vi "Dashboard Main.vi"() -> ()   [LabVIEW 2023]
uses:
  52f2dcef-b32f-41dc-9262-467f65fbdc6c.vi
  <vilib>/Rock Robotics/Network Tables/NT Write String Array.vi
  <vilib>/Rock Robotics/WPI/Dashboard/WPI_DashboardLogging Global.vi
  <vilib>/Rock Robotics/Network Tables/NT Write Boolean.vi
panel:
  in  "Camera Settings Right":T1={"Frame Rate"=30, "Compression"=30, "Size"=1, "DB Camera Config"=FALSE} {"Frame Rate" scale=1.0..30.0; "Compression" scale=100.0..-1.0; "Size" items=["640x480", "320x240", "160x120"]}
  in  "Camera Name Right":string(combo)="No Camera Selection"
  out "NT Connection":bool
  in  "Camera Settings":T1={"Frame Rate"=30, "Compression"=30, "Size"=1, "DB Camera Config"=FALSE} {"Frame Rate" scale=1.0..30.0; "Compression" scale=100.0..-1.0; "Size" items=["640x480", "320x240", "160x120"]}
  in  "Camera Name":string(combo)="No Camera Selection"
  in  "TCP":refnum<k5>
  in  "Rec Mode":enum32{"Stop", "Record", "Playback"}(radio)
  out "Robot IP":string
  out "Image Message":string="Timeout in Camera Communications"
  in  "Dashboard Tab":T2(tab)
  in  "Auto Type":string
  out "Match Safe?":bool
  out "Cascade Level":string
  in  "Auto Delay?":bool
  in  "Delay Time (s)":dbl
  out "E.E. Setpoint":dbl
  in  "Aquitaine File":string
  in  "Climb Arm Reset":bool
  out "Intake Setpoint":dbl
  in  "Auto Calibrate":bool=TRUE
  in  "Robot Selector":u16(ring) items=["2468 Competition", "2468 Practice"]
  in  "Manual Paths":string[](array[string])
  in  "Max Rotation":dbl=400.0
  in  "Max Translation":dbl=19.0
  in  "Deadband":dbl=0.05
  in  "Auto Selector":T3(ring)
  out "IMU":dbl(knob) scale=-180.0..180.0
  in  "Select Auto":string(combo)="Select Autonomous ..."
  out "Mode":T4(ring)=enum."Auto Disabled"
  out "Camera Perf":cluster{"Bandwidth (Mbps)":dbl, "FPS":dbl}
  out "Cascade Sensor":dbl
  out "Camera Perf 2":string
  out "Auto Picture":picture
  out "Cascade State":string
  out "Has Coral?":string
  out "Algae State":string
  out "Climb State":string
  in  "Amp Scale":dbl=0.97
  out "Shooter Hood":dbl
  out "Distance from Speaker":dbl
  out "Trap Auto Align":bool
  out "Camera Image Right":T5(plugin-control)
  out "Speaker Auto Align":bool
  out "Field Centric":bool
  out "Camera Image":T5(plugin-control)
  out "Current Shot":T6(ring)
  out "In Range?":bool
  out "Tree":string(tree)
  # "HW"
  # "HW"
  # "IMU"
  # "SWERVE"
  # "AUTONOMOUS"
  # "CONFIGS"
  # "FEEDBACK"
  # "INTAKE VIEW"
  # "SHOOTER VIEW"
  # "FIELD CENTRIC"
  # "SPEAKER AA"
  # "TRAP AA"
  # "CAN ERROR"
  # "SENSOR FAULT"
  # "GATE DRIVER"
  # "No POWER"
  # "FuLL FORWARD"
  # "FuLL REVERSE"
  # "BRUSHED BRAKE"
  # "BRUSHED COAST"
  # "BRUSHLESS BRAKE"
  # "BRUSHLESS COAST"
  # "RECOVERY MODE/OFF"
  # "https://cdn8.bigcommerce.com/s-t3eo8vwp22/product_images/uploaded_images/fault-no-12v.gif"
  # "PIGEON 2"
  # "DAMAGED HARDWARE"
  # "BOOTLOADER"
  # "CAN FAULT"
  # "ROBOT DISABLED"
  # "ROBOT ENABLED"
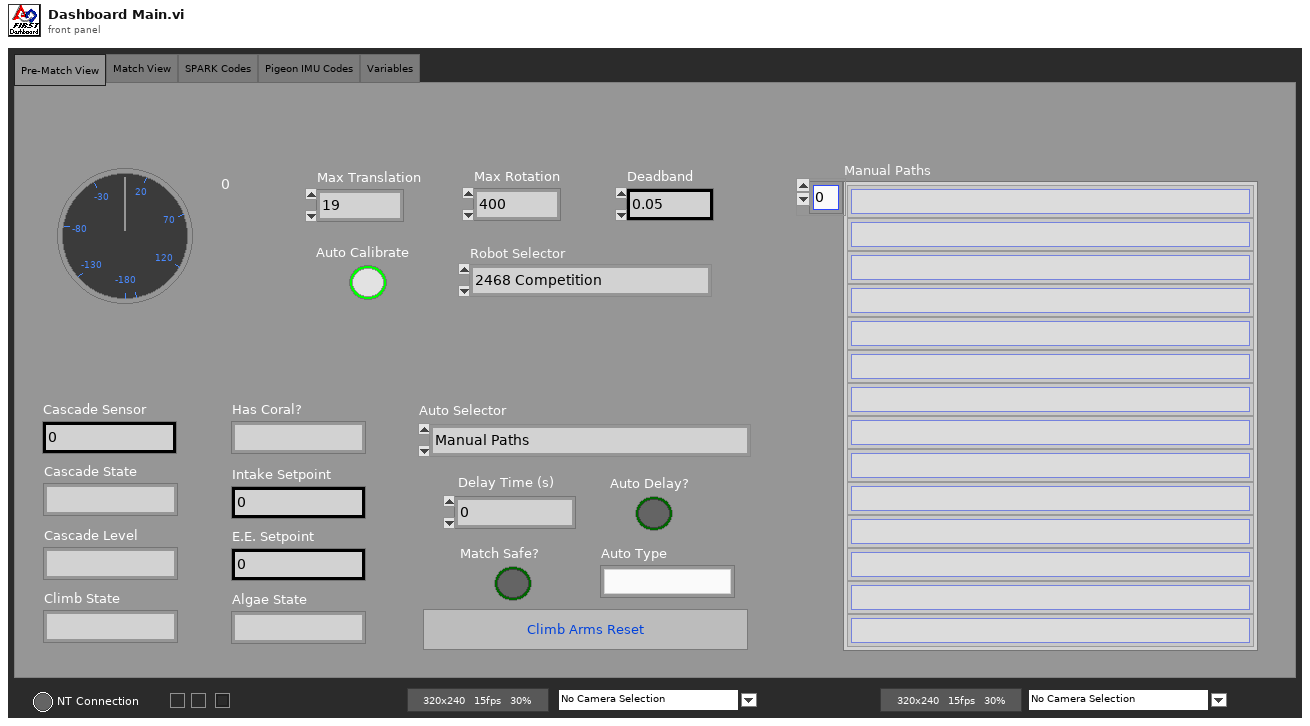
[diagram p1: front panel]
types:
  T1 = cluster{"Frame Rate":i32, "Compression":i32, "Size":u16, "DB Camera Config":bool}
  T2 = enum32{"Pre-Match View", "Match View", "SPARK Codes", "Pigeon IMU Codes", "Variables"}
  T3 = enum16{"Manual Paths", "Reef Align Auto", "1 High Coral Left Side", "1 High Coral Center (SAFE)"}
  T4 = enum8{"Tele-Op Disabled", "Tele-Op Enabled", "Auto Disabled", "Auto Enabled", "Test Disabled", "Test Enabled", "Disconnected", "No Code", "E-Stop"}
  T5 = typedef "IMAQ Image.ctl" = refnum<image>
  T6 = enum32{"Soft Lob", "Amp", "Subwoofer", "Long Lob", "Idle", "Zero", "Trap", "Interpolation"}
  T7 = cluster{"Save Path":path, "Interval (s)":dbl, "Keep":i32}
  T8 = typedef "Image Type" = u32
  T9 = enum32{"Pre-Match View", "Match View", "SparkMax Codes", "Pigeon IMU Codes", "Variables"}
  T10 = cluster{"IDs":cluster{"RPC field ID":u16, "Unique ID":u16}, "String":string}
  T11 = cluster{"Dashboard Tab":refnum<vi>, "Rec Mode":refnum<vi>, "Tree":refnum<vi>, "Camera Perf 2":refnum<vi>, "Camera Settings":refnum<vi>, "Camera Name":refnum<vi>, "Camera Image":refnum<vi>}
  T12 = cluster{"Global Rectangle":i32[], "Contours":cluster{"Contour Type":u32, "ROI Type":u32, "Points":i32[]}[]}
  T13 = cluster{"Camera Name Right":string, string, "Saved DB Images Info":cluster{"Save Path":path, "Interval (s)":dbl, "Keep":i32}}
  T14 = cluster{"Camera Name":string, string, "Saved DB Images Info":cluster{"Save Path":path, "Interval (s)":dbl, "Keep":i32}}
  T15 = cluster{"Error Strings":string, "Disable Counts":cluster{u16, u16}, "Rail Faults":cluster{u16, u16, u16}, "Robot IP":string, "DB Mode":u8, "Event Info":cluster{"Name":string, "Type":u8, "Number":u16, "Replay":u8}}
  T16 = cluster{"Storage":cluster{"Disk Free":u64, "RAM Block":u32, "RAM free":u32}, "CPU Utilization":cluster{"CPU % ISR":sgl, "CPU % Time Crit":sgl, "CPU % Timed Str":sgl, "CPU % High":sgl, "CPU % Above":sgl, "CPU % Normal":sgl, "CPU % Low":sgl}, "CAN":cluster{"% Bus Utilization":sgl, "Bus Off Cnt":u32, "TX_FIFO Full Cnt":u32, "Receive Error Cnt":u8, "Transmit Error Cnt":u8}, "HID":cluster{"HID Outputs":u32, "Rumble Low":u16, "Rumble High":u16}[]}
  T17 = cluster{"Status bits":cluster{"Test Mode":bool, "Autonomous":bool, "Enabled":bool, "Code Start":bool, "Brownout":bool, "Reserved 2":bool, "Reserved 3":bool, "E-Stop":bool}, "Code Trace":cluster{"Disabled":bool, "TeleOp":bool, "Auto":bool, "Test":bool}, "Controller Type":enum16{"unknown", "cRIO", "roboRio"}, "Code?":enum16{"unknown", "noCode", "code"}, "Battery V":dbl}
  T18 = cluster{"Control Bits":cluster{"TestMode":bool, "Autonomous":bool, "Enabled":bool, "FMS Present":bool, bool, bool, bool, "E-Stop":bool}, "Team Station ":u8, "Countdown":sgl, "Joystick Values":cluster{"Axes":dbl[], "Buttons":bool[], "POVs":i16[]}[]}
  T19 = typedef "imagedata.ctl" = cluster{"image type":i32, "image depth":i32, "image":u8[], "mask":u8[], "colors":u32[], "Rectangle":cluster{"left":i16, "top":i16, "right":i16, "bottom":i16}}
  T20 = cluster{"Operation":enum16{"Update", "Clear"}, "Color Box":u32}[]
  T21 = cluster{"Image Size":bool, "Image Type":bool, "Pixel Value":bool, "ROI Information":bool, "Zoom Factor":bool}
  T22 = cluster{"Shift":bool, "Ctrl":bool, "Alt":bool, "Cmd":bool, "Opt":bool}
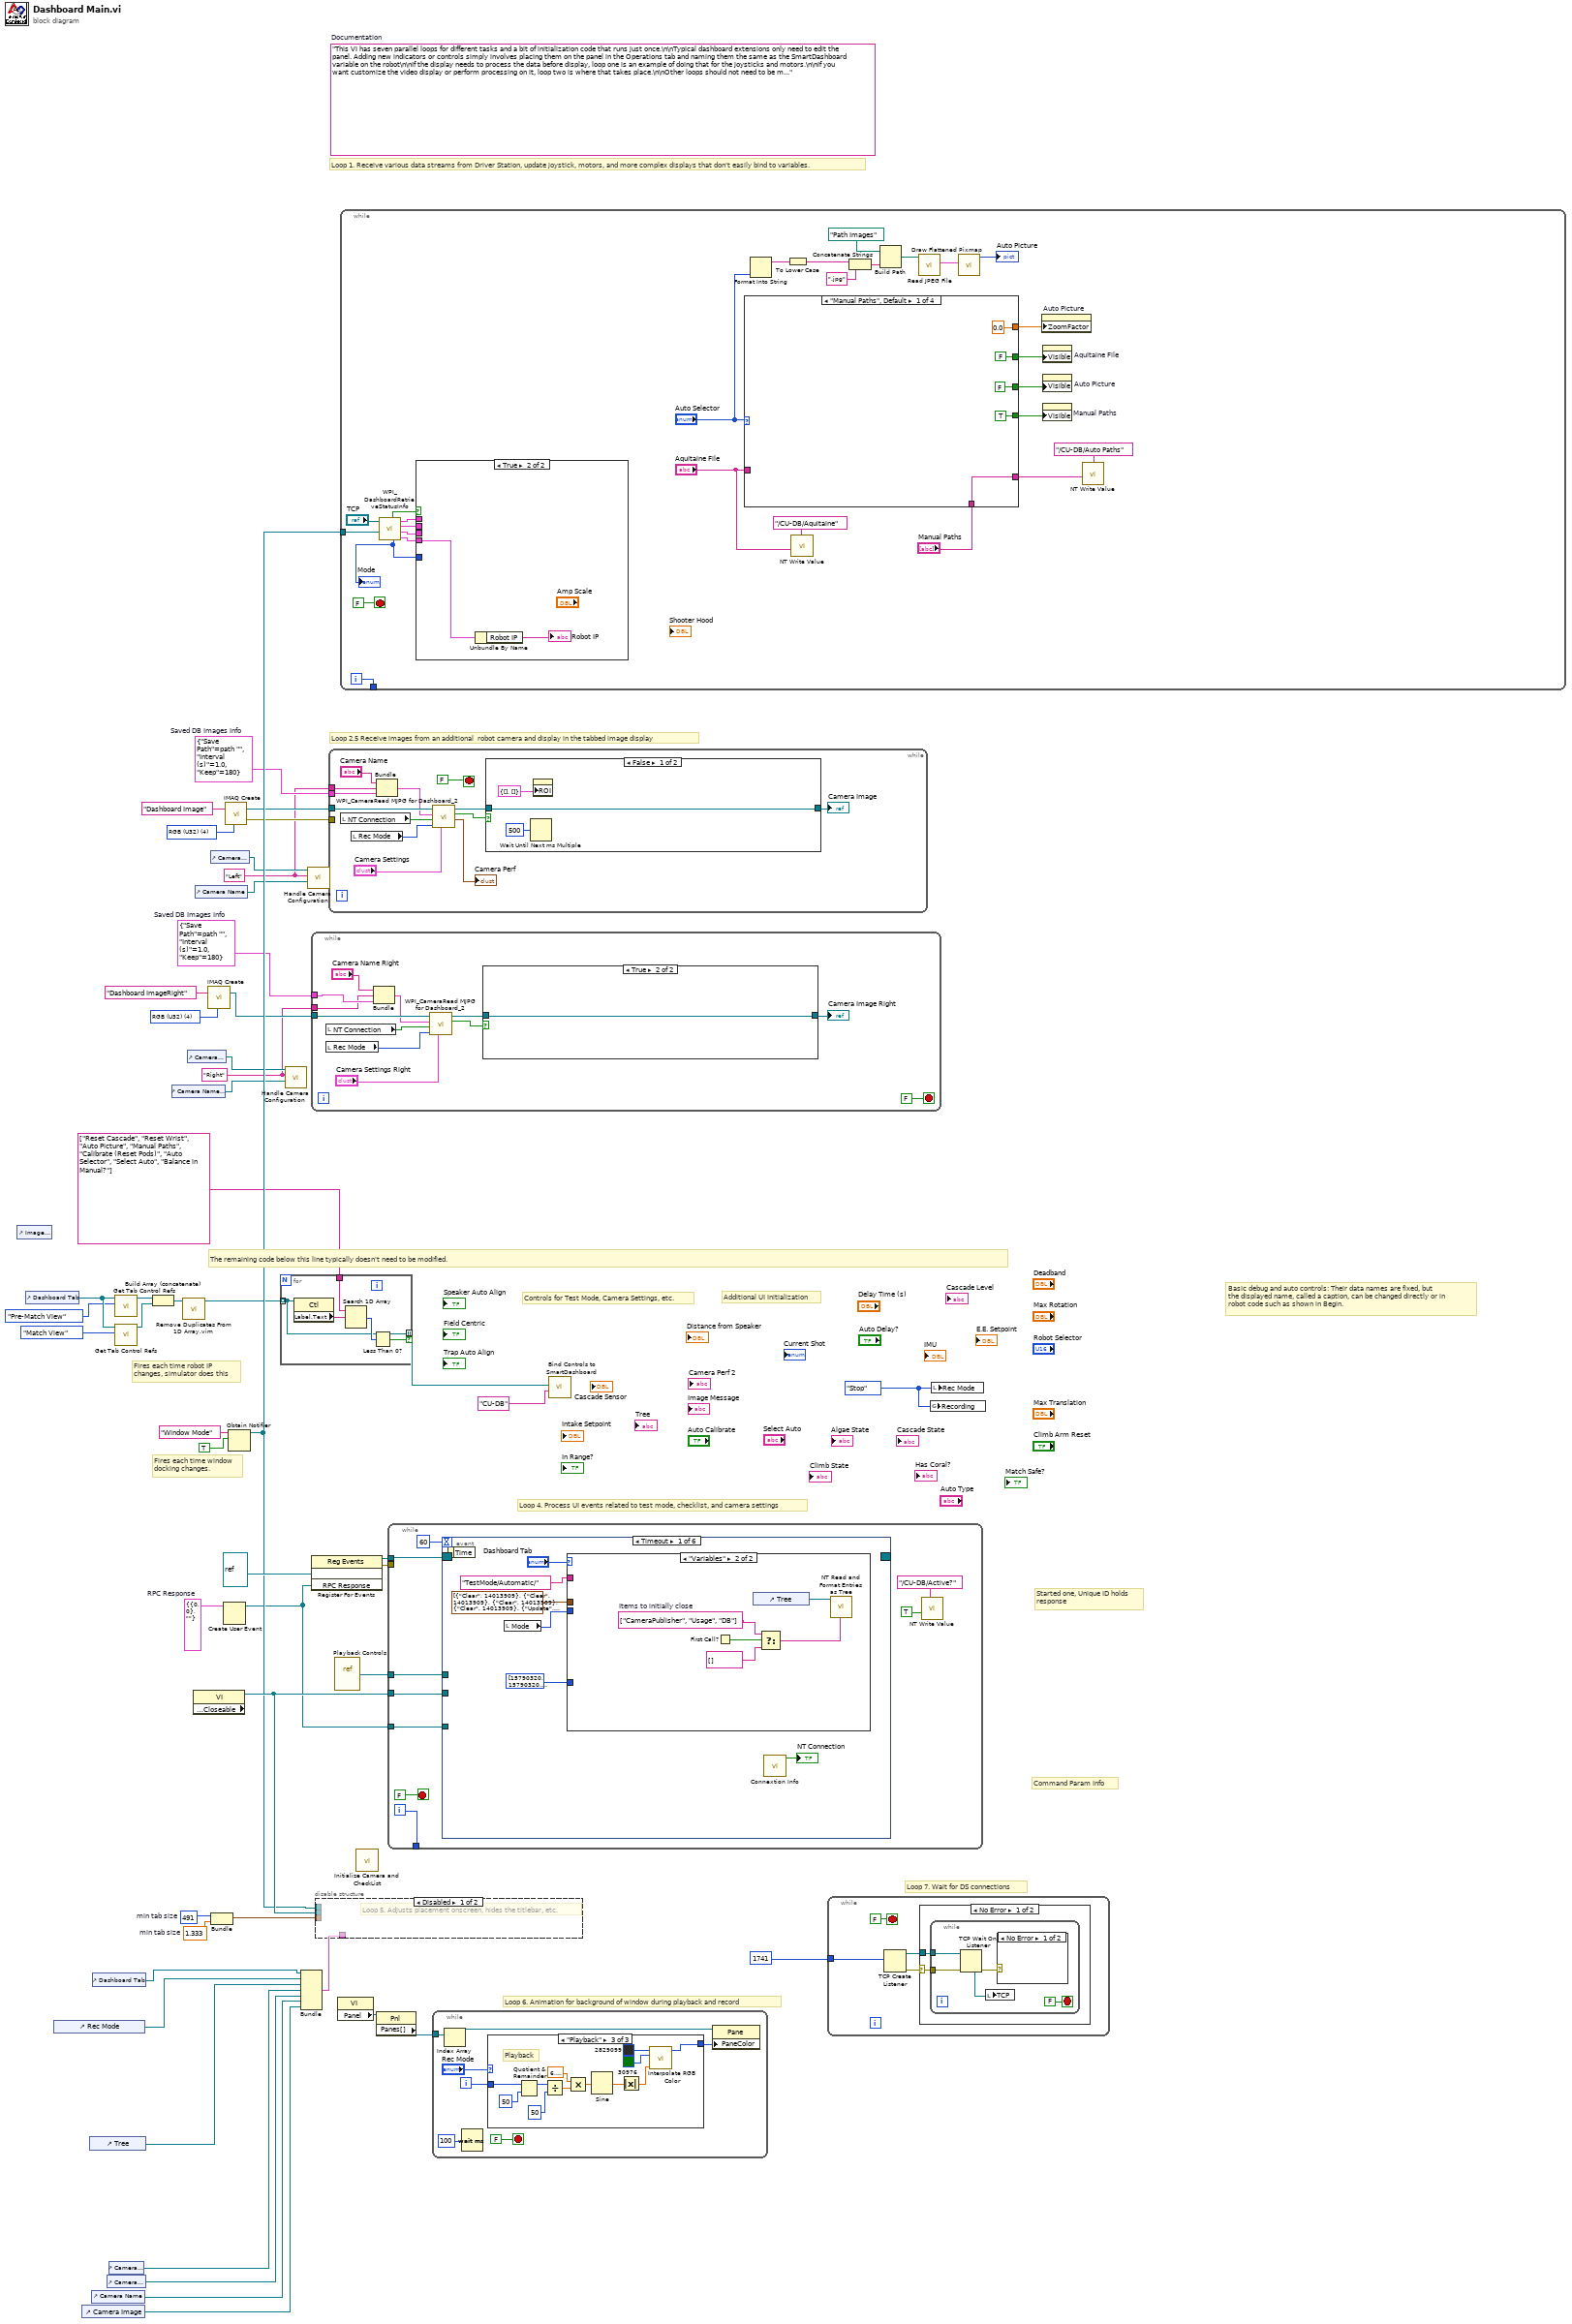
[diagram p0: block diagram]
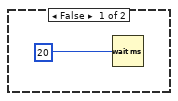
[diagram p2: hidden frame]
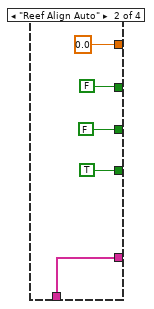
[diagram p3: hidden frame]
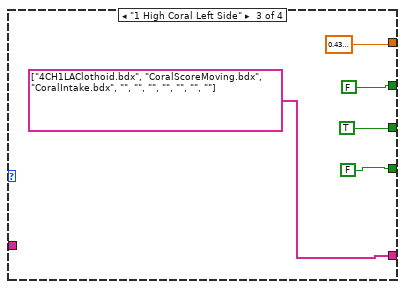
[diagram p4: hidden frame]
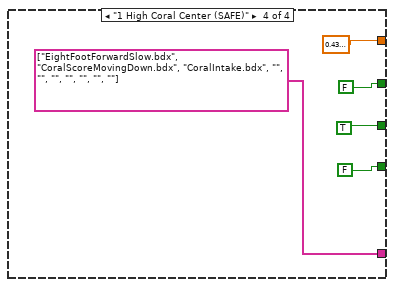
[diagram p5: hidden frame]
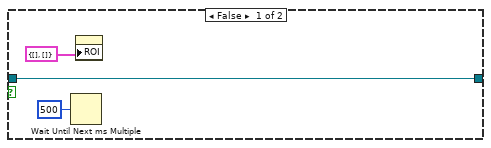
[diagram p8: hidden frame]
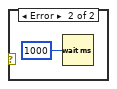
[diagram p9: hidden frame]
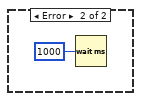
[diagram p10: hidden frame]
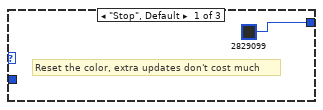
[diagram p11: hidden frame]
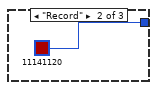
[diagram p12: hidden frame]
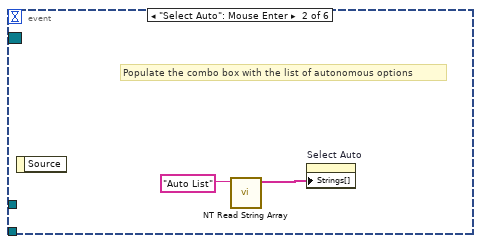
[diagram p14: hidden frame]
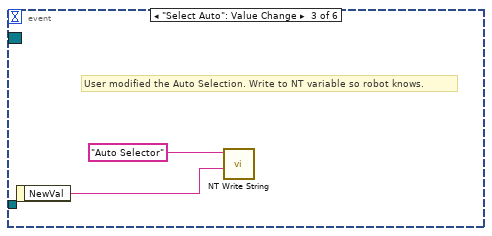
[diagram p15: hidden frame]
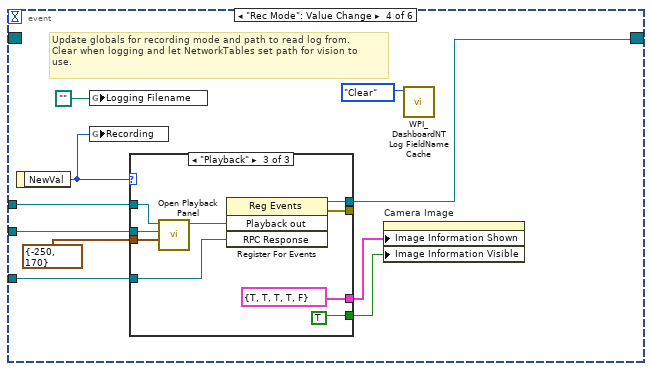
[diagram p16: hidden frame]
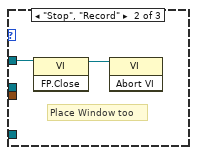
[diagram p18: hidden frame]
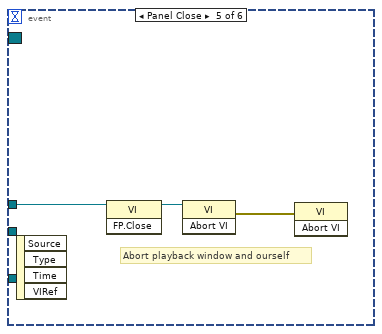
[diagram p19: hidden frame]
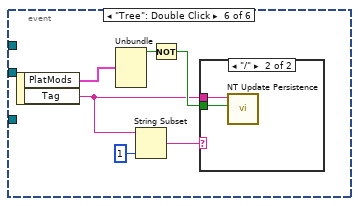
[diagram p20: hidden frame]
diagram:
  w1 = "Right"
  w6 = T7 {"Save Path"=path "", "Interval (s)"=1.0, "Keep"=180}  # Saved DB Images Info
  w8 = T8 4 items=["Grayscale (U8)", "Grayscale (I16)", "Grayscale (SGL)", "Complex (CSG)", "RGB (U32)", "HSL (U32)", "RGB (U64)"] ("Image Type")
  w24 = T7 {"Save Path"=path "", "Interval (s)"=1.0, "Keep"=180}  # Saved DB Images Info
  w5 = "Left"
  w29 = T8 4 items=["Grayscale (U8)", "Grayscale (I16)", "Grayscale (SGL)", "Complex (CSG)", "RGB (U32)", "HSL (U32)", "RGB (U64)"] ("Image Type")
  w33 = T10 {"IDs"={"RPC field ID"=0, "Unique ID"=0}, "String"=""}  # RPC Response
  w40 = 491  # min tab size
  w39 = 1.333  # min tab size
  w42 = enum32{"Stop", "Record", "Playback"}."Stop" ("Rec Mode")
  (unwired) "This VI has seven parallel loops for different tasks and a bit of initialization code that runs just once.\n\nTypical dashboard extensions only need to edit the panel. Adding new indicators or controls simply involves placing them on the panel in the Operations tab and naming them the same as the SmartDashboard variable on the robot\n\nIf the display needs to process the data before display, loop one is an example of doing that for the joysticks and motors.\n\nIf you want customize the video display or perform processing on it, loop two is where that takes place.\n\nOther loops should not need to be modified. They are pretty standard, and document the task they perform."  # Documentation
  # "Loop 2.5 Receive images from an additional  robot camera and display in the tabbed image display"
  # "Command Param Info"
  # "Started one, Unique ID holds\nresponse"
  # "Loop 7. Wait for DS connections"
  # "Basic debug and auto controls: Their data names are fixed, but\nthe displayed name, called a caption, can be changed directly or in\nrobot code such as shown in Begin."
  # "Controls for Test Mode, Camera Settings, etc."
  # "Additional UI Initialization"
  # "Loop 6. Animation for background of window during playback and record"
  # "Fires each time robot IP\nchanges, simulator does this"
  # "Fires each time window\ndocking changes."
  # "The remaining code below this line typically doesn't need to be modified."
  # "Loop 4. Process UI events related to test mode, checklist, and camera settings"
  # "Loop 1. Receive various data streams from Driver Station, update joystick, motors, and more complex displays that don't easily bind to variables."
  n1 = control-ref of="Image Message"() -> ()  [unwired: 1 out]
  n2 = control-ref of="Dashboard Tab"() -> (w22:refnum<vi>)
  n3 = control-ref of="Rec Mode"() -> (w36:refnum<vi>)
  n4 = control-ref of="Camera Image"() -> (w25:refnum<vi>)
  n5 = control-ref of="Tree"() -> (w23:refnum<vi>)
  n6 = control-ref of="Camera Name"() -> (w26:refnum<vi>)
  n7 = control-ref of="Dashboard Tab"() -> (w14:refnum<vi>)
  n8 = control-ref of="Camera Settings"() -> (w27:refnum<vi>)
  n9 = control-ref of="Camera Perf 2"() -> (w31:refnum<vi>)
  n10 = call <vilib>:"Get Tab Control Refs.vi"("Page Index"=T9."Pre-Match View" ("Dashboard Tab"), "TabControl in"=w22) -> ("ControlsOnPage"=w21:refnum<vi>[])  [unwired: 9 in]
  n11 = call <vilib>:"Get Tab Control Refs.vi"("Page Index"=T9."Match View" ("Dashboard Tab"), "TabControl in"=w22) -> ("ControlsOnPage"=w20:refnum<vi>[])  [unwired: 9 in]
  n12 = Build Array (concatenate)(w21, w20) -> (w19:refnum<vi>[])
  n13 = control-ref of="Camera Name Right"() -> (w2:refnum<vi>)
  n14 = call "Remove Duplicates From 1D Array.vim"("array"=w19) -> ("array with duplicates removed"=w16:refnum<vi>[])  [unwired: 10 in]
  n15 = control-ref of="Camera Settings Right"() -> (w3:refnum<vi>)
  n16 = property class="VI" props=["Front Panel.Closeable"]() -> (reference out=w41:refnum<vi>)  [unwired: 2 in, 2 out]
  n17 = control-ref of="Camera Name"() -> (w10:refnum<vi>)
  n18 = call "IMAQ Create"("Image Name"="Dashboard ImageRight", "Image Type"=w8) -> ("New Image"=w4:T5)  [unwired: 2 in, 2 out]
  n19 = control-ref of="Camera Settings"() -> (w11:refnum<vi>)
  n20 = Bundle("min tab size"=w40, "min tab size"=w39) -> (w38:cluster{"min tab size":i32, "min tab size":dbl})  [unwired: 1 in]
  n21 = Create User Event(user event datatype=w33) -> (user event=w32:refnum<user-event>)  [unwired: 1 in, 1 out]
  n22 = call "IMAQ Create"("Image Name"="Dashboard Image", "Image Type"=w29) -> ("New Image"=w9:T5, "error out"=w28:errorcluster)  [unwired: 2 in, 1 out]
  n23 = Obtain Notifier(name (unnamed)="Window Mode", notification data type=TRUE) -> (notifier out=w35:refnum<notifier>)  [unwired: 2 in, 2 out]
  n24 = for {
    tunnel: string[] ["Reset Cascade", "Reset Wrist", "Auto Picture", "Manual Paths", "Calibrate (Reset Pods)", "Auto Selector", "Select Auto", "Balance in Manual?"] -> [w56]
    tunnel: w16 -> [w53] mode=indexing
    tunnel: [w53] -> w15 mode=indexing if=w52
    n25 = property class="Ctl"(reference=w53) -> ("Label.Text"=w55:string)  [unwired: 1 in, 2 out]
    n26 = Search 1D Array(1D array=w56, element=w55) -> (index of element=w54:i32)  [unwired: 1 in]
    n27 = Less Than 0?(x=w54) -> (x < 0?=w52:bool)
  }
  n28 = call "Handle Camera Configuration.vi"("CameraNameRef"=w2, "Display Name"=w1, "ClusterRef"=w3) -> ()  [unwired: 9 in]
  n29 = Bundle("Dashboard Tab"=w14, "Rec Mode"=w36, "Tree"=w23, "Camera Perf 2"=w31, "Camera Settings"=w27, "Camera Name"=w26, "Camera Image"=w25) -> (w37:T11)  [unwired: 1 in]
  n30 = call "Handle Camera Configuration.vi"("CameraNameRef"=w10, "Display Name"=w5, "ClusterRef"=w11) -> ()  [unwired: 9 in]
  n31 = while {
    tunnel: w6 -> [w61]
    tunnel: w4 -> [w64]
    tunnel: w1 -> [w58]
    stop <- FALSE stop-if-true
    n32 = local read "NT Connection"() -> (w63:bool)
    n33 = local read "Rec Mode"() -> (w62:enum32{"Stop", "Record", "Playback"})
    n34 = Bundle("Camera Name Right"="Camera Name Right", w58, "Saved DB Images Info"=w61) -> (w57:T13)  [unwired: 1 in]
    n35 = call <vilib>:"WPI_CameraRead MJPG for Dashboard_2.vi"("Camera Settings"="Camera Settings Right", "Rec Mode"=w62, "NT Connection"=w63, "Capture Info"=w57, "Image in"=w64) -> ("Active"=w66:bool, "Image\\ out"=w67:T5)  [unwired: 4 in, 1 out]
    n36 = case shown="True" w66 {
      tunnel: w67 -> [w70 w72]
      tunnel: [w70 w72] -> w68
      frame False {
        n37 = Wait Until Next ms Multiple(millisecond multiple=u32 500) -> ()  [unwired: 1 out]
        n38 = property on="Camera Image" class="ImageControl"("ROI"=T12 {"Global Rectangle"=[], "Contours"=[]}) -> ()  [unwired: 2 in, 2 out]
      }
      frame True {
      }
    }
    "Camera Image Right" <- w68
  }
  n39 = register-events(refnum<vi> refnum, w32) -> (reference out=w45:refnum<event-registration>, error out=w44:errorcluster)  [unwired: 2 in]
  n40 = disable-structure shown="Disabled" {
    disable-tunnel: w41 -> [_ _]
    disable-tunnel: w38 -> [_ _]
    disable-tunnel: w37 -> [_ _]
    disable-tunnel: w35 -> [_ _]
    frame Disabled {
      # "Loop 5. Adjusts placement onscreen, hides the titlebar, etc."
    }
    frame Enabled {
    }
  }
  n41 = while {
    tunnel: w9 -> [w85]
    tunnel: w28 -> [_]
    tunnel: w24 -> [w74]
    tunnel: w5 -> [w76]
    stop <- FALSE stop-if-true
    n42 = local read "NT Connection"() -> (w75:bool)
    n43 = local read "Rec Mode"() -> (w73:enum32{"Stop", "Record", "Playback"})
    n44 = Bundle("Camera Name"="Camera Name", w76, "Saved DB Images Info"=w74) -> (w79:T14)  [unwired: 1 in]
    n45 = call <vilib>:"WPI_CameraRead MJPG for Dashboard_2.vi"("Camera Settings"="Camera Settings", "Rec Mode"=w73, "NT Connection"=w75, "Capture Info"=w79, "Image in"=w85) -> ("perf info"=→"Camera Perf":cluster{"Bandwidth (Mbps)":dbl, "fps":dbl}, "Active"=w81:bool, "Image\\ out"=w83:T5)  [unwired: 4 in]
    n46 = case shown="False" w81 {
      tunnel: w83 -> [w87 w89]
      tunnel: [w87 w89] -> w80
      frame False {
        n47 = Wait Until Next ms Multiple(millisecond multiple=u32 500) -> ()  [unwired: 1 out]
        n48 = property on="Camera Image" class="ImageControl"("ROI"=T12 {"Global Rectangle"=[], "Contours"=[]}) -> ()  [unwired: 2 in, 2 out]
      }
      frame True {
      }
    }
    "Camera Image" <- w80
  }
  n49 = vi-ref "Playback Controls.vi"() -> (w46:refnum<vi>)
  n50 = property class="VI"() -> ("Panel"=w48:refnum<vi>)  [unwired: 2 in, 2 out]
  n51 = while {
    tunnel: [w116] -> _
    tunnel: w35 -> [w109]
    i -> [w116]
    stop <- FALSE stop-if-true
    n52 = call <vilib>:"WPI_DashboardRetrieveStatusInfo.vi"("Window Mode Notifier"=w109, "TCP Cnx"="TCP") -> ("Power and Errors"=w111:T15, "Robot Metrics"=w114:T16, "Status Info"=w115:T17, "Control Info"=w112:T18, "Robot Mode"=w93:T4, "Process?"=w113:bool)  [unwired: 4 in]
    "Mode" <- w93
    n53 = case shown="True" w113 {
      tunnel: w115 -> [_ _]
      tunnel: w114 -> [_ _]
      tunnel: w112 -> [_ _]
      tunnel: w111 -> [_ w120]
      tunnel: w93 -> [_ _]
      frame False {
        n54 = Wait (ms)(milliseconds to wait=u32 20) -> ()  [unwired: 1 out]
      }
      frame True {
        n55 = Unbundle By Name(w120) -> ("Robot IP"=→"Robot IP":string)
      }
    }
    n56 = case shown="\"Manual Paths\", Default" "Auto Selector" {
      tunnel: [w121 w126 string[] ["4CH1LAClothoid.bdx", "CoralScoreMoving.bdx", "CoralIntake.bdx", "", "", "", "", "", "", ""] ("Manual Paths") string[] ["EightFootForwardSlow.bdx", "CoralScoreMovingDown.bdx", "CoralIntake.bdx", "", "", "", "", "", "", ""] ("Manual Paths")] -> w90
      tunnel: [FALSE ("Visible") FALSE ("Visible") TRUE ("Visible") TRUE ("Visible")] -> w108
      tunnel: [TRUE ("Visible") TRUE ("Visible") FALSE ("Visible") FALSE ("Visible")] -> w95
      tunnel: [FALSE ("Visible") FALSE ("Visible") FALSE ("Visible") FALSE ("Visible")] -> w105
      tunnel: "Aquitaine File" -> [_ _ _ _]
      tunnel: [sgl 0.0 ("Zoom Factor") sgl 0.0 ("Zoom Factor") sgl 0.44 ("Zoom Factor") sgl 0.44 ("Zoom Factor")] -> w92
      tunnel: "Manual Paths" -> [w121 w126 _ _]
      frame "Manual Paths", Default {
      }
      frame "Reef Align Auto" {
      }
      frame "1 High Coral Left Side" {
      }
      frame "1 High Coral Center (SAFE)" {
      }
    }
    n57 = Format Into String("Auto Selector") -> (resulting string=w99:string)  [unwired: 3 in, 1 out]
    n58 = To Lower Case(string=w99) -> (all lower case string=w100:string)
    n59 = call-poly <vilib>:"NT Write Value.vi"("value"="Aquitaine File", "name"="/CU-DB/Aquitaine") -> ()  [unwired: 9 in, 1 out]
    n60 = Concatenate Strings(w100, ".jpg" ("string")) -> (w101:string)
    n61 = Build Path(base path=path "Path Images", name or relative path=w101) -> (appended path=w104:path)
    n62 = call <vilib>:"Read JPEG File.vi"("path to JPEG file"=w104) -> ("image data"=w103:T19)  [unwired: 8 in, 2 out]
    n63 = call <vilib>:"Draw Flattened Pixmap.vi"("image data"=w103) -> ("new picture"=→"Auto Picture":picture)  [unwired: 8 in]
    n64 = property on="Auto Picture" class="Pict"("ZoomFactor"=w92) -> ()  [unwired: 2 in, 2 out]
    n65 = property on="Aquitaine File" class="Str"("Visible"=w105) -> ()  [unwired: 2 in, 2 out]
    n66 = property on="Auto Picture" class="Pict"("Visible"=w108) -> ()  [unwired: 2 in, 2 out]
    n67 = property on="Manual Paths" class="Arr (strict)"("Visible"=w95) -> ()  [unwired: 2 in, 2 out]
    n68 = call-poly <vilib>:"NT Write Value.vi"("value"=w90, "name"="/CU-DB/Auto Paths") -> ()  [unwired: 9 in, 1 out]
  }
  n69 = call "Initialize Camera and CheckList.vi"() -> ()  [unwired: 12 in]
  n70 = property class="Pnl"(reference=w48) -> ("Panes[]"=w49:refnum<vi>[])  [unwired: 1 in, 2 out]
  n71 = while {
    tunnel: [w147] -> _
    tunnel: w46 -> [w146]
    tunnel: w45 -> [w145]
    tunnel: w44 -> [_]
    tunnel: w41 -> [w144]
    tunnel: w32 -> [w143]
    i -> [w147]
    stop <- FALSE stop-if-true
    n72 = event shown="[0] Timeout" {
      selector: w145 -> [_ _ _ _ _ _]
      dyn-events: [_ _ _ w171 _ _] -> _
      timeout: u32 60 ("milliseconds to wait") -> [_ _ _ _ _ _]
      tunnel: w146 -> [_ _ _ w173 w188 _]
      tunnel: w144 -> [_ _ _ w169 _ _]
      tunnel: w143 -> [_ _ _ w167 _ _]
      event Timeout {
        n73 = event-data() -> ()  [unwired: 1 in, 1 out]
        n74 = local read "Mode"() -> (w152:T4)
        n75 = case shown="\"Variables\"" "Dashboard Tab" {
          tunnel: "TestMode/Automatic/" ("Name Pattern") -> [_ _]
          tunnel: T20 [{"Operation"=enum."Clear", "Color Box"=14013909}, {"Operation"=enum."Clear", "Color Box"=14013909}, {"Operation"=enum."Clear", "Color Box"=14013909}, {"Operation"=enum."Clear", "Color Box"=14013909}, {"Operation"=enum."Update", "Color Box"=14013909}, {"Operation"=enum."Update", "Color Box"=16777215}, {"Operation"=enum."Clear", "Color Box"=14013909}, {"Operation"=enum."Clear", "Color Box"=14013909}, {"Operation"=enum."Clear", "Color Box"=14013909}] -> [_ _]
          tunnel: w152 -> [_ _]
          tunnel: u32[] [15790320, 15790320, 15790320, 15790320, 16777215, 16777215, 15790320, 15790320, 15790320] -> [_ _]
          frame Default {
          }
          frame "Variables" {
            w158 = string[] ["CameraPublisher", "Usage", "DB"]  # Items to initially close
            n76 = First Call?() -> (First Call?: T/F=w159:bool)
            n77 = control-ref of="Tree"() -> (w160:refnum<vi>)
            n78 = Select(t=w158, s=w159, f=string[] []) -> (s? t:f=w156:string[])
            n79 = call <vilib>:"NT Read and Format Entries as Tree.vi"("Tags to  Close"=w156, "Tree Refnum"=w160) -> ()  [unwired: 8 in, 2 out]
          }
        }
        n80 = call <vilib>:"Connextion Info.vi"() -> ("Connected"=→"NT Connection":bool)  [unwired: 10 in, 1 out]
      }
      event "Select Auto": Mouse Enter {
        # "Populate the combo box with the list of autonomous options"
        n81 = event-data() -> ()  [unwired: 1 in, 1 out]
        n82 = call <vilib>:"NT Read String Array.vi"("name"="Auto List" ("Name")) -> ("value"=w161:string[])  [unwired: 8 in, 2 out]
        n83 = property on="Select Auto" class="CmbBox"("Strings[]"=w161) -> ()  [unwired: 2 in, 2 out]
      }
      event "Select Auto": Value Change {
        # "User modified the Auto Selection. Write to NT variable so robot knows."
        n84 = event-data() -> ("NewVal"=w163:string)  [unwired: 1 in]
        n85 = call <vilib>:"NT Write String.vi"("value"=w163, "name"="Auto Selector" ("Name")) -> ()  [unwired: 9 in, 1 out]
      }
      event "Rec Mode": Value Change {
        # "Update globals for recording mode and path to read log from.\nClear when logging and let NetworkTables set path for vision to\nuse."
        n86 = event-data() -> ("NewVal"=w174:enum32{"Stop", "Record", "Playback"})  [unwired: 1 in]
        n87 = global write "WPI_DashboardLogging Global.vi" "Logging Filename"(path "") -> ()
        n88 = global write "WPI_DashboardLogging Global.vi" "Recording"(w174) -> ()
        n89 = case shown="\"Playback\"" w174 {
          tunnel: w173 -> [_ w176 w185]
          tunnel: [_ _ w184] -> w171
          tunnel: [_ _ w183] -> _
          tunnel: w169 -> [_ _ w181]
          tunnel: cluster{i32, i32} {-250, 170} -> [_ _ w180]
          tunnel: [_ _ T21 {"Image Size"=TRUE, "Image Type"=TRUE, "Pixel Value"=TRUE, "ROI Information"=TRUE, "Zoom Factor"=FALSE} ("Image Information Shown:All Elements")] -> w165
          tunnel: [_ _ TRUE ("Zoom Factor")] -> w166
          tunnel: w167 -> [_ _ w177]
          frame Default {
          }
          frame "Stop", "Record" {
            # "Place Window too"
            n90 = invoke class="VI" method="FP.Close"(reference=w176) -> (reference out=w175:refnum<vi>)  [unwired: 2 in, 2 out]
            n91 = invoke class="VI" method="Abort VI"(reference=w175) -> ()  [unwired: 2 in, 3 out]
          }
          frame "Playback" {
            n92 = call "Open Playback Panel.vi"("Offset"=w180, "DB VI Ref"=w181, "Playback in"=w185) -> ("Playback out"=w182:refnum<vi>)  [unwired: 8 in]
            n93 = register-events(w182, w177) -> (reference out=w184:refnum<event-registration>, error out=w183:errorcluster)  [unwired: 2 in]
          }
        }
        n94 = property on="Camera Image" class="ImageControl"("Image Information Shown"=w165, "Image Information Visible"=w166) -> ()  [unwired: 2 in, 2 out]
        n95 = call <vilib>:"WPI_DashboardNT Log FieldName Cache.vi"("Operation"=enum16{"Lookup/Add", "Index", "Clear"}."Clear") -> ()  [unwired: 8 in, 3 out]
      }
      event Panel Close {
        # "Abort playback window and ourself"
        n96 = event-data() -> ()  [unwired: 1 in, 4 out]
        n97 = invoke class="VI" method="FP.Close"(reference=w188) -> (reference out=w187:refnum<vi>)  [unwired: 2 in, 2 out]
        n98 = invoke class="VI" method="Abort VI"(reference=w187) -> (error out=w186:errorcluster)  [unwired: 2 in, 2 out]
        n99 = invoke class="VI" method="Abort VI"(error in=w186) -> ()  [unwired: 2 in, 3 out]
      }
      event "Tree": Double Click {
        n100 = event-data() -> ("PlatMods"=w194:T22, "Tag"=w191:string)  [unwired: 1 in]
        n101 = Unbundle(w194) -> ("Shift"=w193:bool)  [unwired: 4 out]
        n102 = String Subset(string=w191, length (rest)=1 ("length (rest)")) -> (substring=w190:string)  [unwired: 1 in]
        n103 = Not(x=w193) -> (.not. x?=w192:bool)
        n104 = case shown="\"/\"" w190 {
          tunnel: w191 -> [_ w196]
          tunnel: w192 -> [_ w195]
          frame Default {
          }
          frame "/" {
            n105 = call <vilib>:"NT Update Persistence.vi"("Persistence"=w195, "Name"=w196) -> ()  [unwired: 9 in, 1 out]
          }
        }
      }
    }
    n106 = call-poly <vilib>:"NT Write Value.vi"("value"=TRUE ("Boolean"), "name"="/CU-DB/Active?" ("Name")) -> ()  [unwired: 9 in, 1 out]
  }
  n107 = Index Array(array=w49) -> (element=w47:refnum<vi>)  [unwired: 1 in]
  n108 = while {
    tunnel: w47 -> [w198]
    i -> [w201]
    stop <- FALSE stop-if-true
    n109 = Wait (ms)(milliseconds to wait=u32 100) -> ()  [unwired: 1 out]
    n110 = case shown="\"Playback\"" "Rec Mode" {
      tunnel: w201 -> [_ _ w216]
      tunnel: [u32 2829099 ("Base Color") u32 11141120 ("Target Color") w205] -> w197
      frame "Stop", Default {
        # "Reset the color, extra updates don't cost much"
      }
      frame "Record" {
      }
      frame "Playback" {
        # "Playback"
        n111 = Quotient & Remainder(x=w216, y=u32 50 ("milliseconds to wait")) -> (x-y*floor(x/y)=w212:u32)  [unwired: 1 out]
        n112 = Divide(x=w212, y=u32 50 ("milliseconds to wait")) -> (x/y=w209:dbl)
        n113 = Multiply(x=6.283185307179586, y=w209) -> (x*y=w214:dbl)
        n114 = Sine(x=w214) -> (sin(x)=w213:dbl)
        n115 = Absolute Value(x=w213) -> (abs(x)=w206:dbl)
        n116 = call "Interpolate RGB Color.vi"("Proportion"=w206, "Target Color"=u32 30976, "Base Color"=u32 2829099) -> ("Result Color"=w205:u32)  [unwired: 8 in]
      }
    }
    n117 = property class="Pane"(reference=w198, "PaneColor"=w197) -> ()  [unwired: 1 in, 2 out]
  }
  n118 = call <vilib>:"Bind Controls to SmartDashboard.vi"("Path Prefix"="CU-DB", "Bound Control Refs"=w15) -> ()  [unwired: 10 in]
  n119 = while {
    tunnel: u16 1741 ("timeout ms (25000)") -> [w218]
    stop <- FALSE stop-if-true
    n120 = TCP Create Listener(10:w218) -> (0:w217:errorcluster, 3:w219:refnum<k5>)  [unwired: 4 in, 1 out]
    n121 = case shown="No Error" w217 {
      selector: w217 -> [w221 _]
      tunnel: w219 -> [w222 _]
      frame No Error {
        n122 = while {
          tunnel: w222 -> [w225]
          tunnel: w221 -> [w224]
          stop <- FALSE stop-if-true
          n123 = TCP Wait On Listener(8:w224, 11:w225) -> (0:w226:errorcluster, 4:w227:refnum<k5>)  [unwired: 2 in, 3 out]
          n124 = local write "TCP"(w227) -> ()
          n125 = case shown="No Error" w226 {
            frame No Error {
            }
            frame Error {
              n126 = Wait (ms)(milliseconds to wait=u32 1000) -> ()  [unwired: 1 out]
            }
          }
        }
      }
      frame Error {
        n127 = Wait (ms)(milliseconds to wait=u32 1000) -> ()  [unwired: 1 out]
      }
    }
  }
  n128 = global write "WPI_DashboardLogging Global.vi" "Recording"(w42) -> ()
  n129 = local write "Rec Mode"(w42) -> ()
